vi "PSP-Nx-Dual.vi"() -> ()   [LabVIEW 2009]
uses:
  <vilib>/NXT/Subs/LVHSConnector.ctl
  <vilib>/NXT/Block Support/NXT_InputPort.ctl
  mindsensors.com LVEE Toolkit/Dual/PSP-Nx-DM.vi
panel:
  out "Button Status":bool
  in  "Cluster":cluster{"Button to Check":u16} {"Button to Check" items=["Start", "Select", "Up", "Down", "Left", "Right", "^", "[]", "X", "O", "L1", "L2", "L3", "R1", "R2", "R3"]}
  in  "Input Port":T1 items=["Port 1", "Port 2", "Port 3", "Port 4"]
  out "NXT dup":T2={"error"={"status"=FALSE, "code"=0, "source"=""}, "address"="", "NXT #"=-1, "Show Error"=TRUE, "Connection"=4} {"Connection" items=["USB", "Bluetooth", "USB then Bluetooth", "Last Connection", "Preference"]}
  in  "NXT":T2={"error"={"status"=FALSE, "code"=0, "source"=""}, "address"="", "NXT #"=-1, "Show Error"=TRUE, "Connection"=4} {"Connection" items=["USB", "Bluetooth", "USB then Bluetooth", "Last Connection", "Preference"]}
  out "Right Y:":u8=127
  out "Right  X:":u8=128
  out "Left Y":u8=128
  out "Left  X":u8=128
  in  "stop":bool
  # "mindsensors.com\nCopyright (c) 2009 by mindsensors.com\nEmail: info (<at>) mindsensors (<dot>) com\n\nThis program is free software. You can redistribute it and/or modify\nit under the terms of the GNU General Public License as published by\nthe Free Software Foundation; version 3 of the License.\nRead the license at: http://www.gnu.org/licenses/gpl.txt"
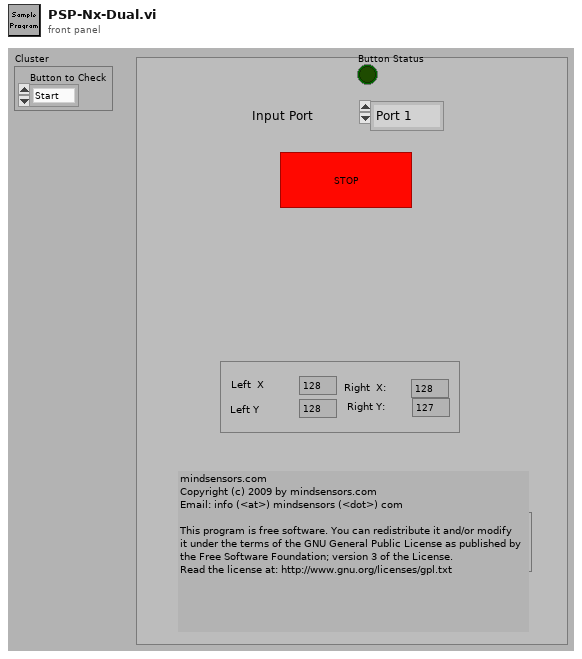
[diagram p1: front panel]
types:
  T1 = typedef "NXT_InputPort.ctl" = u8
  T2 = typedef "LVHSConnector.ctl" = cluster{"error":errorcluster, "address":string, "NXT #":i32, "Show Error":bool, "Connection":u16}
  T3 = cluster{"left x":u8, "left y":u8, "right x":u8, "right y":u8, "button 1":u8, "button 2":u8, "Status of Button Checked\n(pressed or not pressed)":bool}
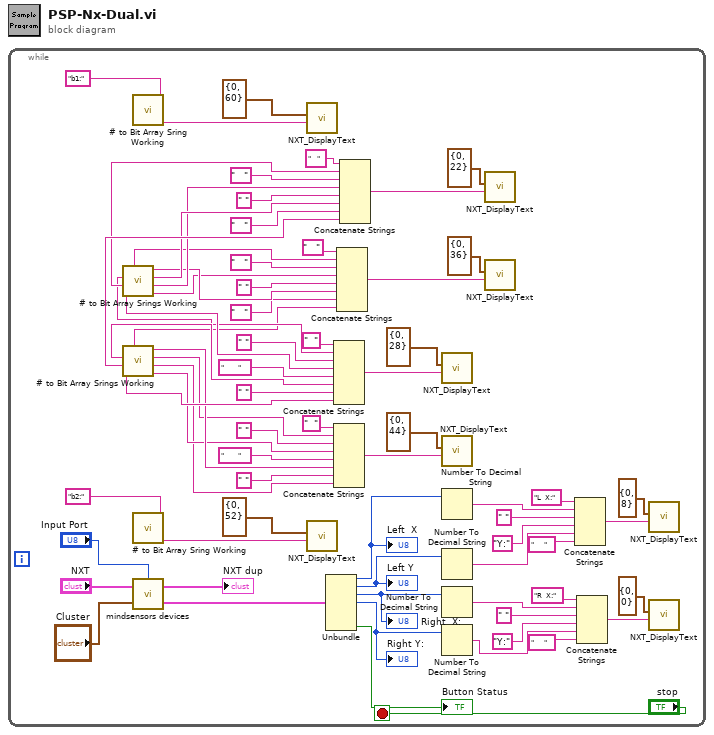
[diagram p0: block diagram]
diagram:
  n1 = while {
    stop <- "stop" stop-if-true
    n2 = call "# to Bit Array Srings Working.vi"() -> ("P1"=w55:string, "P1 2"=w59:string, "P1 3"=w56:string, "P1 4"=w50:string, "P1 5"=w53:string, "P1 6"=w61:string, "P1 7"=w60:string, "P1 8"=w48:string)  [unwired: 3 in]
    n3 = call "# to Bit Array Srings Working.vi"() -> ("P1"=w57:string, "P1 2"=w62:string, "P1 3"=w58:string, "P1 4"=w52:string, "P1 5"=w54:string, "P1 6"=w51:string, "P1 7"=w23:string, "P1 8"=w49:string)  [unwired: 3 in]
    n4 = call "# to Bit Array Sring Working.vi"("Choose String"="b1:") -> ("Final String"=w68:string)  [unwired: 9 in]
    n5 = call "# to Bit Array Sring Working.vi"("Choose String"="b2:") -> ("Final String"=w65:string)  [unwired: 9 in]
    n6 = call-poly "mindsensors devices.vi"("Cluster"="Cluster", "NXT"="NXT", "Input Port"="Input Port") -> ("output cluster"=w70:T3, "NXT dup"=→"NXT dup":T2)
    n7 = call "NXT_DisplayText.vi"("Text"=w68, "Location (0,0)"=cluster{"X":i16, "Y":i16} {"X"=0, "Y"=60}) -> ()  [unwired: 9 in, 1 out]
    n8 = call "NXT_DisplayText.vi"("Text"=w65, "Location (0,0)"=cluster{"X":i16, "Y":i16} {"X"=0, "Y"=52}) -> ()  [unwired: 9 in, 1 out]
    n9 = Unbundle(w70) -> ("left x"=w6:u8, "left y"=w5:u8, "right x"=w4:u8, "right y"=w3:u8, "Status of Button Checked\n(pressed or not pressed)"=→"Button Status":bool)  [unwired: 2 out]
    "Left  X" <- w6
    "Left Y" <- w5
    "Right  X:" <- w4
    "Right Y:" <- w3
    n10 = Concatenate Strings("  " ("string"), w55, " " ("string"), w56, "       " ("string"), w57, " " ("string"), w58) -> (w26:string)
    n11 = Concatenate Strings("  " ("string"), w51, " " ("string"), w49, "       " ("string"), w54, " " ("string"), w23) -> (w38:string)
    n12 = Concatenate Strings("   " ("string"), w50, "   " ("string"), w48, " " ("string"), w53, "   " ("string"), w52) -> (w42:string)
    n13 = Concatenate Strings("   " ("string"), w59, "   " ("string"), w60, " " ("string"), w61, "   " ("string"), w62) -> (w31:string)
    n14 = call "NXT_DisplayText.vi"("Text"=w26, "Location (0,0)"=cluster{"X":i16, "Y":i16} {"X"=0, "Y"=28}) -> ()  [unwired: 9 in, 1 out]
    n15 = call "NXT_DisplayText.vi"("Text"=w38, "Location (0,0)"=cluster{"X":i16, "Y":i16} {"X"=0, "Y"=44}) -> ()  [unwired: 9 in, 1 out]
    n16 = Number To Decimal String(number=w6) -> (decimal integer string=w15:string)  [unwired: 1 in]
    n17 = Number To Decimal String(number=w5) -> (decimal integer string=w8:string)  [unwired: 1 in]
    n18 = Number To Decimal String(number=w4) -> (decimal integer string=w19:string)  [unwired: 1 in]
    n19 = Number To Decimal String(number=w3) -> (decimal integer string=w11:string)  [unwired: 1 in]
    n20 = call "NXT_DisplayText.vi"("Text"=w31, "Location (0,0)"=cluster{"X":i16, "Y":i16} {"X"=0, "Y"=22}) -> ()  [unwired: 9 in, 1 out]
    n21 = call "NXT_DisplayText.vi"("Text"=w42, "Location (0,0)"=cluster{"X":i16, "Y":i16} {"X"=0, "Y"=36}) -> ()  [unwired: 9 in, 1 out]
    n22 = Concatenate Strings("L  X:" ("string"), w15, " " ("string"), "Y:" ("string"), w8, "     " ("string")) -> (w17:string)
    n23 = Concatenate Strings("R  X:" ("string"), w19, " " ("string"), "Y:" ("string"), w11, "     " ("string")) -> (w21:string)
    n24 = call "NXT_DisplayText.vi"("Text"=w17, "Location (0,0)"=cluster{"X":i16, "Y":i16} {"X"=0, "Y"=8}) -> ()  [unwired: 9 in, 1 out]
    n25 = call "NXT_DisplayText.vi"("Text"=w21, "Location (0,0)"=cluster{"X":i16, "Y":i16} {"X"=0, "Y"=0}) -> ()  [unwired: 9 in, 1 out]
  }
